vi "SQL-LV Generate Update Method.vi"(8 "error in (no error)":errorcluster, 9 "SQL-LV Control Paths":T1, 10 "Table Name":string, 11 "Save as":path) -> (0 "error out":errorcluster, 3 "Save as out":path)   [LabVIEW 2021]
uses:
  SQL-LV Table Control Paths.ctl
  edt.lib/vi_script.lib/Control Replacement Param.ctl
  DB Method Enum.ctl
  edt.lib/vi_script.lib/Constant Replacement Param.ctl
  edt.lib/vi_script.lib/Array Item Replacement Param (CTL).ctl
  edt.lib/vi_script.lib/Replace Control in VI (Scalar).vi
  edt.lib/vi_script.lib/Replace Constant in VI (Scalar).vi
  edt.lib/vi_script.lib/EDT VI Script.lvlib
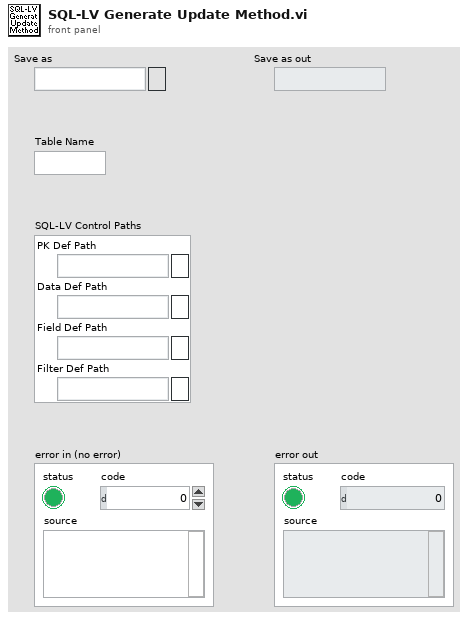
[diagram p1: front panel]
types:
  T1 = typedef "SQL-LV Table Control Paths.ctl" = cluster{"PK Def Path":path, "Data Def Path":path, "Field Def Path":path, "Filter Def Path":path}
  T2 = typedef "EDT VI Script.lvlib/Control Replacement Param.ctl" = cluster{"Placeholder Name":string, "CTL File Path":path, "Indicator":bool}
  T3 = typedef "EDT VI Script.lvlib/Array Item Replacement Param (CTL).ctl" = cluster{"Array Control Name":string, "Item CTL File Path":path}
  T4 = typedef "EDT VI Script.lvlib/Constant Replacement Param.ctl" = cluster{"Label.Text":string, "Value":variant}
  T5 = typedef "DB Method Enum.ctl" = enum16{"Insert", "Delete", "Select", "Update", "List"}
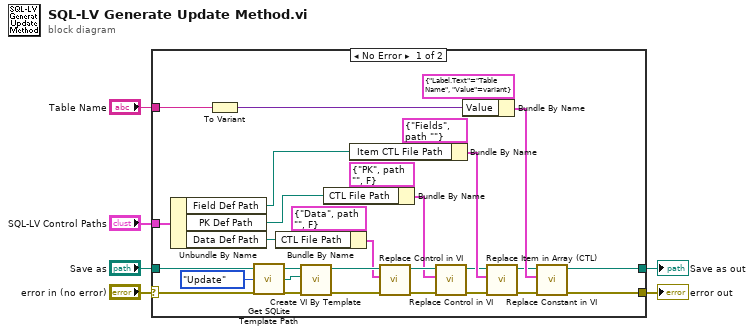
[diagram p0: block diagram]
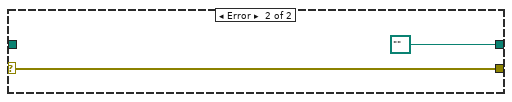
[diagram p2: hidden frame]
diagram:
  n1 = case shown="No Error" "error in (no error)" {
    selector: "error in (no error)" -> [w32 w35]
    tunnel: [w7 path "" ("Save as out")] -> w6
    tunnel: "Save as" -> [w20 _]
    tunnel: [w8 w35] -> w4
    tunnel: "SQL-LV Control Paths" -> [w29 _]
    tunnel: "Table Name" -> [w27 _]
    frame No Error {
      n2 = Unbundle By Name(w29) -> ("Field Def Path"=w23:path, "PK Def Path"=w15:path, "Data Def Path"=w13:path)
      n3 = To Variant(anything=w27) -> (Variant=w26:variant)
      n4 = call "Get SQLite Template Path.vi"("Template Type"=DB_Method_Enum."Update") -> ("Template Path"=w19:path)
      n5 = Bundle By Name(cluster=T2 {"Placeholder Name"="Data", "CTL File Path"=path "", "Indicator"=FALSE} ("Control Replacement Param"), "CTL File Path"=w13) -> (w21:T2)
      n6 = call "Create VI By Template.vi"("error in"=w32, "Template VI Path"=w19, "Save as"=w20) -> ("error out"=w30:errorcluster, "Save as out"=w31:path)  [unwired: 7 in]
      n7 = Bundle By Name(cluster=T2 {"Placeholder Name"="PK", "CTL File Path"=path "", "Indicator"=FALSE} ("Control Replacement Param"), "CTL File Path"=w15) -> (w14:T2)
      n8 = Bundle By Name(cluster=T3 {"Array Control Name"="Fields", "Item CTL File Path"=path ""} ("Array Item Replacement Params"), "Item CTL File Path"=w23) -> (w22:T3)
      n9 = call-poly "Replace Control in VI.vi"("error in"=w30, "Control Replacement Params"=w21, "Original VI"=w31) -> ("error out"=w18:errorcluster, "Save as out"=w17:path)  [unwired: 7 in]
      n10 = call-poly "Replace Control in VI.vi"("error in"=w18, "Control Replacement Params"=w14, "Original VI"=w17) -> ("error out"=w11:errorcluster, "Save as out"=w12:path)  [unwired: 7 in]
      n11 = Bundle By Name(cluster=T4 {"Label.Text"="Table Name", "Value"=variant} ("Constant Replacement Params"), "Value"=w26) -> (w25:T4)
      n12 = call "Replace Item in Array (CTL).vi"("error in"=w11, "Array Item Replacement Params"=w22, "Original VI"=w12) -> ("error out"=w9:errorcluster, "Save as out"=w10:path)  [unwired: 7 in]
      n13 = call-poly "Replace Constant in VI.vi"("error in"=w9, "Constant Replacement Params"=w25, "Original VI"=w10) -> ("error out"=w8:errorcluster, "Save as out"=w7:path)  [unwired: 7 in]
    }
    frame Error {
    }
  }
  "Save as out" <- w6
  "error out" <- w4
